vi "loading.vi"(8 "error in (no error)":errorcluster caption="错误输入（无错误）", 11 "值":refnum<vi>) -> (0 "error out":errorcluster caption="错误输出")   [LabVIEW 2016]
uses:
  <vilib>/Utility/miscctls.llb/LVPointTypeDef.ctl
panel:
  out "进度条":u8(slide) scale=0.0..100.0
  out "下拉列表":u16(ring)
  # "加载中，请稍后......"
  # "Launching..."
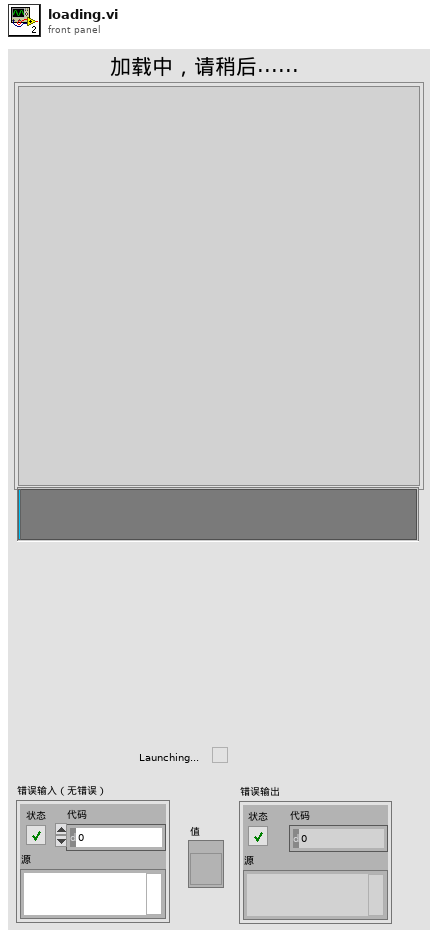
[diagram p1: front panel]
types:
  T1 = typedef "LVPointTypeDef.ctl" = cluster{"Horizontal":i16, "Vertical":i16}
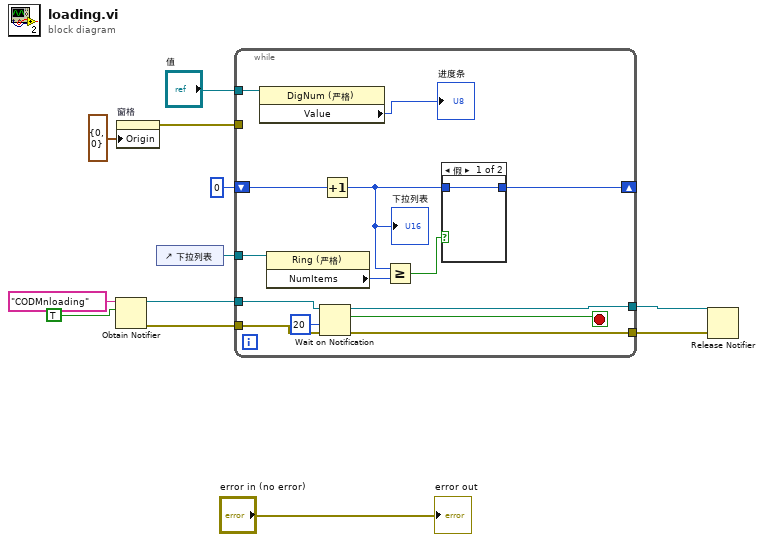
[diagram p0: block diagram]
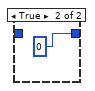
[diagram p2: hidden frame]
diagram:
  n1 = Obtain Notifier(name (unnamed)="CODMnloading" ("名称（未命名）"), notification data type=TRUE) -> (notifier out=w9:refnum<notifier>, error out=w8:errorcluster)  [unwired: 2 in, 1 out]
  n2 = property on="窗格" class="Pane"("Origin"=T1 {"Horizontal"=0, "Vertical"=0} ("原点")) -> (error out=w2:errorcluster)  [unwired: 2 in, 1 out]
  n3 = control-ref of="下拉列表"() -> (w11:refnum<vi>)
  n4 = while {
    shift-right: [w23] -> _
    shift-left: u16 0 -> [w26]
    tunnel: w11 -> [w25]
    tunnel: w9 -> [w20]
    tunnel: w8 -> [w19]
    tunnel: [w16] -> w5
    tunnel: [w15] -> w4
    tunnel: w2 -> [_]
    tunnel: "值" -> [w14]
    stop <- w17 stop-if-true
    n5 = property class="DigNum (严格)"(reference=w14) -> ("Value"=→"进度条":i32)  [unwired: 1 in, 2 out]
    n6 = property class="Ring (严格)"(reference=w25) -> ("NumItems"=w24:u32)  [unwired: 1 in, 2 out]
    n7 = Wait on Notification(notifier=w20, timeout in ms (-1)=20 ("超时毫秒(-1)"), error in (no error)=w19) -> (notifier out=w16:refnum<notifier>, notification=w17:bool, error out=w15:errorcluster)  [unwired: 1 in, 1 out]
    n8 = Increment(x=w26) -> (x+1=w21:u16)
    "下拉列表" <- w21
    n9 = Greater Or Equal?(x=w21, y=w24) -> (x >= y?=w22:bool)
    n10 = case shown="假" w22 {
      tunnel: [w27 u16 0] -> w23
      tunnel: w21 -> [w27 _]
      frame False {
      }
      frame True {
      }
    }
  }
  n11 = Release Notifier(notifier=w5, error in (no error)=w4) -> ()  [unwired: 1 in, 3 out]
  "error out" <- "error in (no error)"
